vi "List Role Policies.vi"(8 "error in (no error)":errorcluster, 10 "Role":string, 11 "IAM Session in":refnum<class "IAM Session.lvclass">) -> (0 "error out":errorcluster, 2 "Role Policies":string[](array[string]), 3 "IAM Session out":refnum<class "IAM Session.lvclass">)   [LabVIEW 2015, in "NI_AWS_IAM.lvlib" / "IAM Session.lvclass"]
uses:
  IAM Session.lvclass
  Core/HTTP Request/Request Options.ctl
  Core/HTTP Request/Name Value Pair.ctl
  Core/HTTP Request/Region handling.ctl
  Core/HTTP Request/URL formatting.ctl
  Core/HTTP Request/HTTP Request.lvclass
  XML Parsing/NI_XML Parsing.lvlib
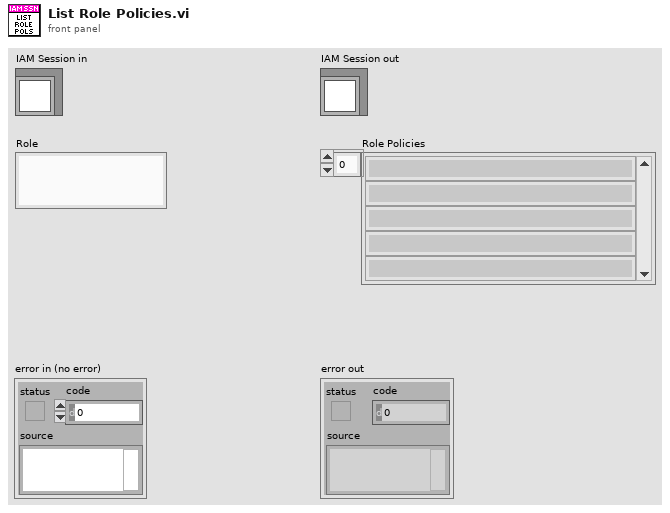
[diagram p1: front panel]
types:
  T1 = typedef "NI_AWS_Core.lvlib/HTTP Request.lvclass/Name Value Pair.ctl" = cluster{"name":string, "value":string}
  T2 = typedef "NI_AWS_Core.lvlib/HTTP Request.lvclass/Request Options.ctl" = cluster{"request headers":T1[], "request parameters":T1[], "request body":string, "region handling":T3, "URL formatting":T4}
  T3 = typedef "NI_AWS_Core.lvlib/HTTP Request.lvclass/Region handling.ctl" = enum16{"use region everywhere", "use region (authentication only)", "use region (URL only)", "ignore region everwhere"}
  T4 = typedef "NI_AWS_Core.lvlib/HTTP Request.lvclass/URL formatting.ctl" = enum16{"region-", "region."}
  T5 = typedef "NI_AWS_Core.lvlib/HTTP Request.lvclass/Response.ctl" = cluster{"Headers":string, "Body":string}
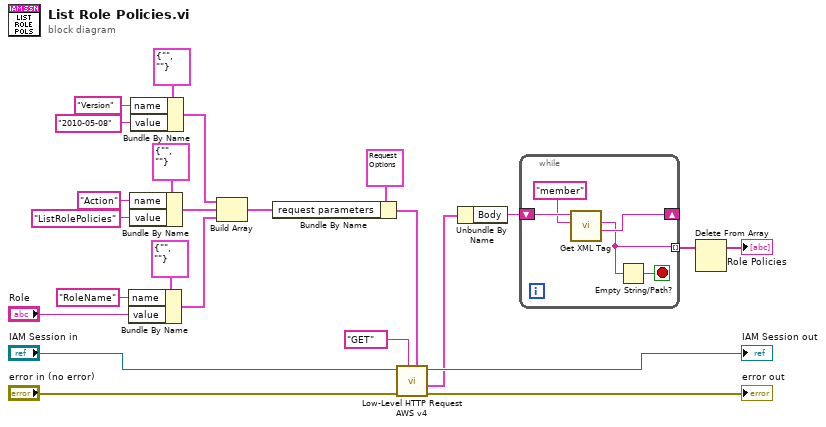
[diagram p0: block diagram]
diagram:
  n1 = Bundle By Name(cluster=T1 {"name"="", "value"=""} ("Name Value Pair"), "name"="RoleName", "value"="Role") -> (w10:T1)
  n2 = Bundle By Name(cluster=T1 {"name"="", "value"=""} ("Name Value Pair"), "name"="Action", "value"="ListRolePolicies") -> (w15:T1)
  n3 = Bundle By Name(cluster=T1 {"name"="", "value"=""} ("Name Value Pair"), "name"="Version", "value"="2010-05-08") -> (w5:T1)
  n4 = Build Array(w5, w15, w10) -> (w14:T1[])
  n5 = Bundle By Name(cluster=T2 {"request headers"=[], "request parameters"=[], "request body"="", "region handling"=enum."use region everywhere", "URL formatting"=enum."region."} ("Request Options"), "request parameters"=w14) -> (w19:T2)
  n6 = call "Low-Level HTTP Request AWS v4.vi"("Request Options"=w19, "HTTP-Verb"="GET", "error in (no error)"="error in (no error)", "AWS Core in"="IAM Session in") -> ("error out"=→"error out":errorcluster, "Response"=w4:T5, "AWS Core out"=→"IAM Session out":refnum<class "IAM Session.lvclass">)  [unwired: 4 in, 1 out]
  n7 = Unbundle By Name(w4) -> ("Body"=w3:string)
  n8 = while {
    shift-right: [w27] -> _
    shift-left: w3 -> [w29]
    tunnel: [w25] -> w2 mode=indexing
    stop <- w26 stop-if-true
    n9 = call "Get XML Tag.vi"("Tag name"="member", "XML String in"=w29) -> ("Remaining string"=w27:string, "Tag value"=w25:string)  [unwired: 5 in, 3 out]
    n10 = Empty String/Path?(string/path=w25) -> (empty?=w26:bool)
  }
  n11 = Delete From Array(array=w2) -> (array with subset deleted=→"Role Policies":string[])  [unwired: 2 in, 1 out]
